vi "Connection Siemens CPU.vi"(8 "error in (no error)":errorcluster, 11 "Siemens Ctr in":T2) -> (0 "error out":errorcluster, 2 "semaphore":T1, 3 "Siemens Ctr out":T2)   [LabVIEW 2014, in "Simatic S7.lvlib"]
uses:
  Simatic S7.lvlib
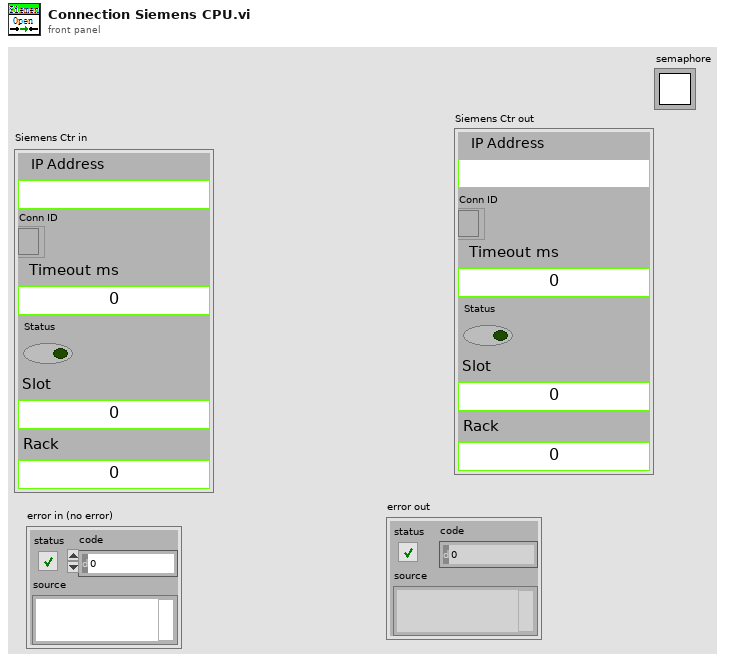
[diagram p1: front panel]
types:
  T1 = typedef "Semaphore RefNum" = refnum<k1>
  T2 = typedef "Simatic S7.lvlib/Siemens Ref.ctl" = cluster{"IP Address ":string, "Conn ID":refnum<k5>, "Timeout ms":i32, "Status":bool, "Slot":u16, "Rack":u16}
  T3 = enum16{"Standard", "Buffered", "CRLF", "Immediate"}
  T4 = typedef "Simatic S7.lvlib/Operation Siemens Ref.ctl" = enum16{"Init", "Add Ref", "Get Ref", "Set Error", "Close Close"}
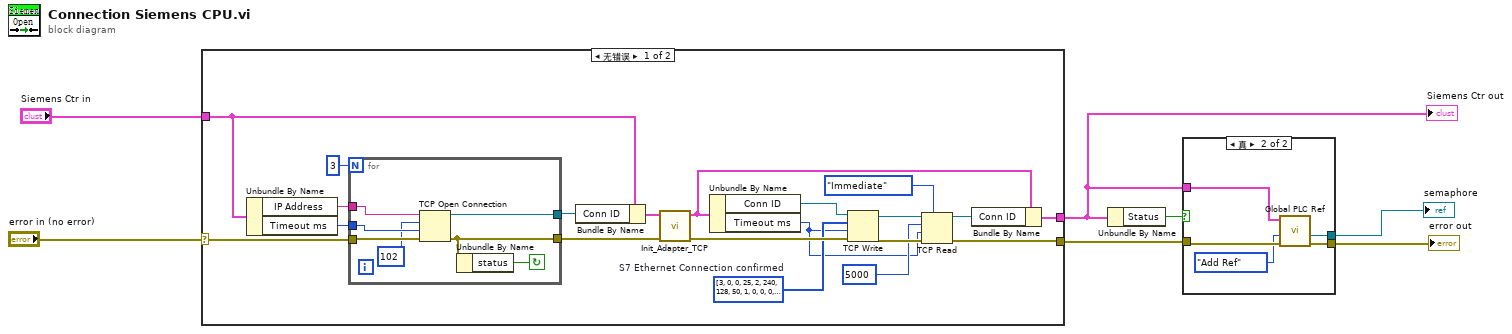
[diagram p0: block diagram]
diagram:
  n1 = case shown="无错误" "error in (no error)" {
    selector: "error in (no error)" -> [w27 w36]
    tunnel: "Siemens Ctr in" -> [w12 w35]
    tunnel: [w10 w36] -> w4
    tunnel: [w9 w35] -> w3
    frame No Error {
      w18 = u8[] [3, 0, 0, 25, 2, 240, 128, 50, 1, 0, 0, 0, 13, 0, 8, 0, 0, 240, 0, 0, 1, 0, 1, 0, 240]  # S7 Ethernet Connection confirmed
      n2 = Unbundle By Name(w12) -> ("IP Address"=w25:string, "Timeout ms"=w24:i32)
      n3 = for {
        N: 3 -> [_]
        tunnel: w27 -> [w34]
        tunnel: w25 -> [w33]
        tunnel: w24 -> [w32]
        tunnel: [w30] -> w22
        tunnel: [w28] -> w23
        stop <- w29 continue-if-true
        n4 = TCP Open Connection(address=w33, remote port or service name=u16 102, timeout ms (60000)=w32, error in (no error)=w34) -> (connection ID=w28:refnum<k5>, error out=w30:errorcluster)  [unwired: 1 in]
        n5 = Unbundle By Name(w30) -> ("status"=w29:bool)
      }
      n6 = Bundle By Name(cluster=w12, "Conn ID"=w23) -> (w21:T2)
      n7 = call "Init_Adapter_TCP.vi"("error in (no error)"=w22, "Siemens Ctr in"=w21) -> ("error out"=w20:errorcluster, "Siemens Ctr out"=w8:T2)  [unwired: 8 in]
      n8 = Unbundle By Name(w8) -> ("Conn ID"=w19:refnum<k5>, "Timeout ms"=w14:i32)
      n9 = TCP Write(connection ID=w19, data in=w18, error in (no error)=w20, 9:w14) -> (connection ID out=w16:refnum<k5>, error out=w17:errorcluster)  [unwired: 1 out]
      n10 = TCP Read(connection ID=w16, bytes to read=5000, error in (no error)=w17, 7:T3."Immediate" ("mode (standard)"), 9:w14) -> (connection ID out=w11:refnum<k5>, error out=w10:errorcluster)  [unwired: 1 out]
      n11 = Bundle By Name(cluster=w8, "Conn ID"=w11) -> (w9:T2)
    }
    frame Error {
    }
  }
  "Siemens Ctr out" <- w3
  n12 = Unbundle By Name(w3) -> ("Status"=w5:bool)
  n13 = case shown="真" w5 {
    tunnel: w4 -> [w37 w42]
    tunnel: w3 -> [_ w41]
    tunnel: [w37 w39] -> w2
    tunnel: [_ w38] -> w1
    frame False {
    }
    frame True {
      n14 = call "Global PLC Ref.vi"("error in (no error)"=w42, "Operation Siemens Ref"=Operation_Siemens_Ref."Add Ref", "Siemens Ctr"=w41) -> ("error out"=w39:errorcluster, "semaphore"=w38:T1)  [unwired: 4 in, 3 out]
    }
  }
  "error out" <- w2
  "semaphore" <- w1
